vi "map_coordinates_xi_zero.vi"(5 "b":dbl, 7 "a":dbl, 8 "Error In":errorcluster, 9 "phi_in":dbl, 10 "xi":dbl, 11 "Parameters":T1) -> (0 "Error Out":errorcluster, 2 "b_pixel":dbl, 3 "a_pixel":dbl)   [LabVIEW 2019]
uses:
  parameters_cluster_typedef.ctl
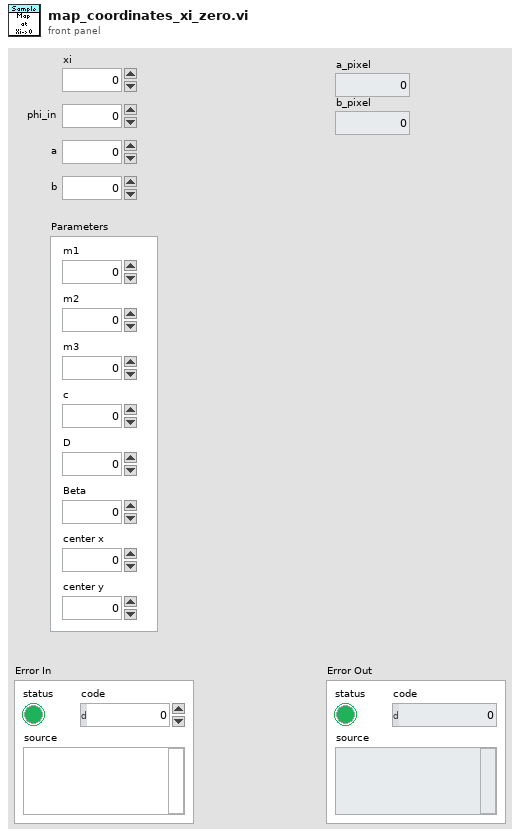
[diagram p1: front panel]
types:
  T1 = typedef "parameters_cluster_typedef.ctl" = cluster{"m1":dbl, "m2":dbl, "m3":dbl, "c":dbl, "D":dbl, "Beta":dbl, "center x":dbl, "center y":dbl}
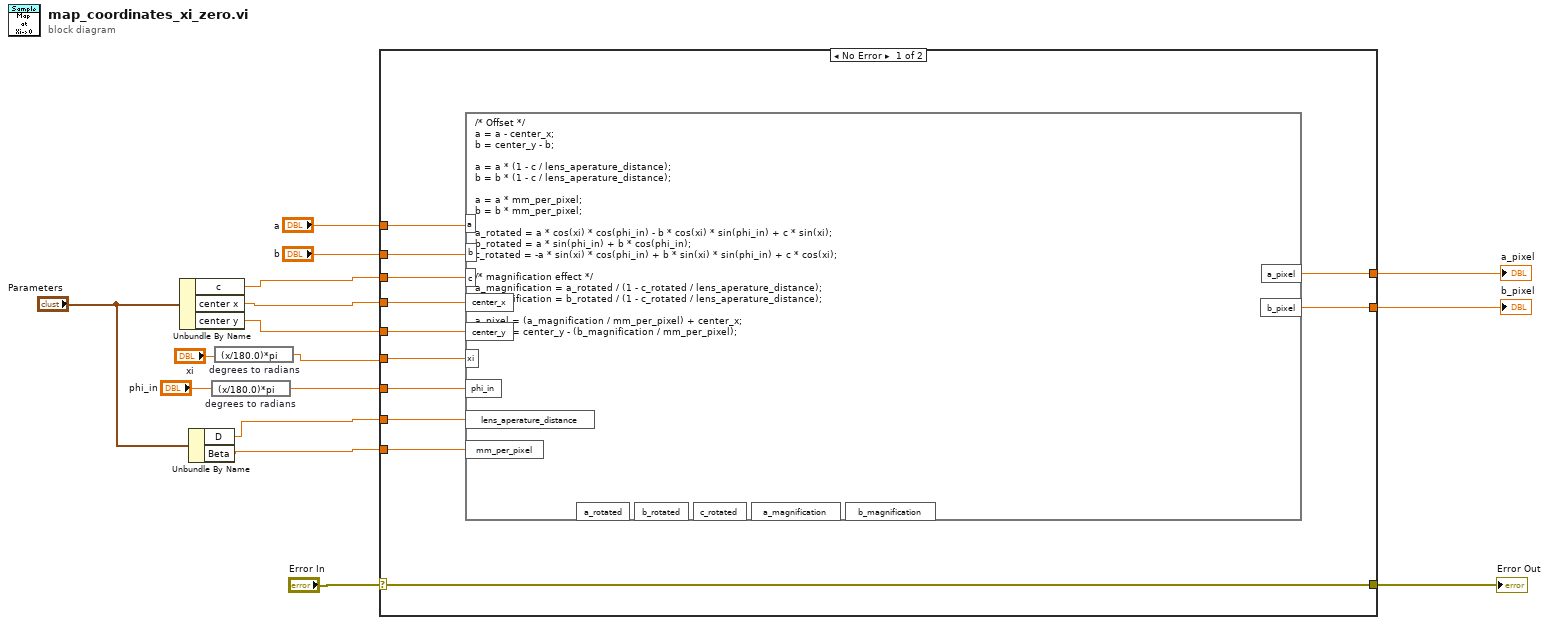
[diagram p0: block diagram]
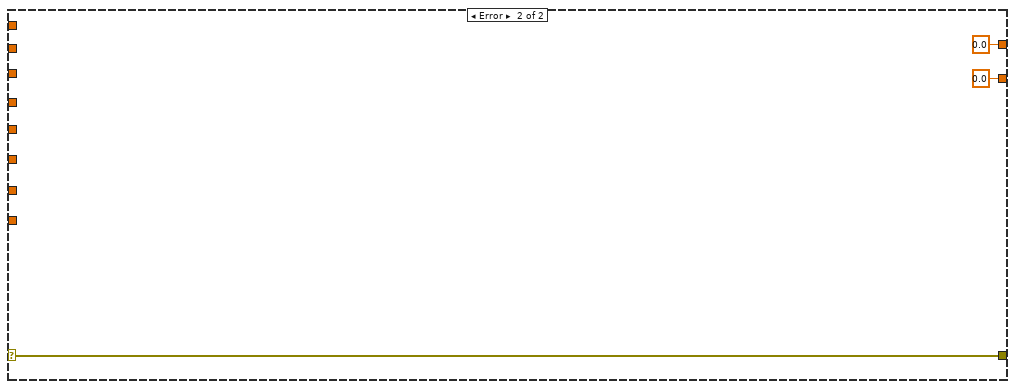
[diagram p2: hidden frame]
diagram:
  n1 = Unbundle By Name("Parameters") -> ("c"=w10:dbl, "center x"=w9:dbl, "center y"=w8:dbl)
  n2 = Unbundle By Name("Parameters") -> ("D"=w6:dbl, "Beta"=w7:dbl)
  n3 = expression code="(x/180.0)*pi" "degrees to radians"("phi_in") -> (w13:dbl)
  n4 = expression code="(x/180.0)*pi" "degrees to radians"("xi") -> (w1:dbl)
  n5 = case shown="No Error" "Error In" {
    selector: "Error In" -> [w17 w31]
    tunnel: "b" -> [w28 _]
    tunnel: "a" -> [w27 _]
    tunnel: w13 -> [w26 _]
    tunnel: [w25 0.0 ("a_pixel")] -> w12
    tunnel: [w24 0.0 ("b_pixel")] -> w11
    tunnel: w10 -> [w23 _]
    tunnel: w9 -> [w22 _]
    tunnel: w8 -> [w21 _]
    tunnel: w7 -> [w20 _]
    tunnel: w6 -> [w19 _]
    tunnel: w1 -> [w18 _]
    tunnel: [w17 w31] -> w3
    frame No Error {
      n6 = formula code="/* Offset */\na = a - center_x;\nb = center_y - b;\n    \na = a * (1 - c / lens_aperature_distance);\nb = b * (1 - c / lens_aperature_distance);\n    \na = a * mm_per_pixel;\nb = b * mm_per_pixel;\n    \na_rotated = a * cos(xi) * cos(phi_in) - b * cos(xi) * sin(phi_in) + c * sin(xi);\nb_rotated = a * sin(phi_in) + b * cos(phi_in);\nc_rotated = -a * sin(xi) * cos(phi_in) + b * sin(xi) * sin(phi_in) + c * cos(xi);\n\n/* magnification effect */\na_magnification = a_rotated / (1 - c_rotated / lens_aperature_distance);\nb_magnification = b_rotated / (1 - c_rotated / lens_aperature_distance);\n\na_pixel = (a_magnification / mm_per_pixel) + center_x;\nb_pixel = center_y - (b_magnification / mm_per_pixel);"("a"=w27, "b"=w28, "c"=w23, "center_x"=w22, "center_y"=w21, "xi"=w18, "phi_in"=w26, "lens_aperature_distance"=w19, "mm_per_pixel"=w20) -> ("a_pixel"=w25:dbl, "b_pixel"=w24:dbl)  [unwired: 5 out]
    }
    frame Error {
    }
  }
  "a_pixel" <- w12
  "b_pixel" <- w11
  "Error Out" <- w3
